vi "Pump Pause Selection.vi"(8 "error in (no error)":errorcluster, 11 "Pump Settings In":T1={"Output Device"=enum."Default", "Masterflex"={"VISA resource name"="", "Simulated?"=FALSE, "Pump Number"=0.0, "Reverse?"=FALSE}, "Ismatech"={"VISA resource name"="", "Simulated?"=FALSE, "Pump Number"=0.0, "Reverse?"=FALSE}, "Ismatech 3 Channel Settings"={"VISA resource name"="", "Pump Number"=1, "Channel Number"=0, "Simulated?"=TRUE, "Reverse?"=FALSE}, "VICI Settings"={"VISA resource name"="", "Pump ID"="", "Pump Head Vol"=0.0, "Reverse?"=FALSE, "Simulated?"=FALSE}, "Tacmina Settings"={"Analog DAQ Task"="", "Digital DAQ Task"=""}, "KNF SIMDOS Settings"={"VISA resource name"="", "Simulated?"=FALSE}, "ASIA Pump C"={"ASIA Pump #"=0, "channel"=0, "Simulated"=FALSE}, "FLOM Settings"={"VISA resource name"="", "Simulated?"=FALSE, "Pump Number"=0.0}, "SSI PR/LD Settings"={"VISA resource name"="", "Simulated?"=FALSE}, "SSI P40 Settings"={"VISA resource name"="", "Simulated?"=FALSE}, "Masterflex 75211 Settings"={"Analog DAQ Task"="", "Digital DAQ Task"=""}} {"Ismatech 3 Channel Settings"."Channel Number" min=0 max=3; "Ismatech 3 Channel Settings"."Pump Number" min=1; "Masterflex"."Pump Number" min=1.0 max=20.0 step=1.0; "Ismatech"."Pump Number" min=1.0 max=20.0 step=1.0; "ASIA Pump C"."channel" min=-1 max=1 step=1}) -> (0 "error out":errorcluster, 1 "Connection Error":bool, 3 "Pump Settings Out":T1={"Output Device"=enum."Default", "Masterflex"={"VISA resource name"="", "Simulated?"=FALSE, "Pump Number"=0.0, "Reverse?"=FALSE}, "Ismatech"={"VISA resource name"="", "Simulated?"=FALSE, "Pump Number"=0.0, "Reverse?"=FALSE}, "Ismatech 3 Channel Settings"={"VISA resource name"="", "Pump Number"=1, "Channel Number"=0, "Simulated?"=TRUE, "Reverse?"=FALSE}, "VICI Settings"={"VISA resource name"="", "Pump ID"="", "Pump Head Vol"=0.0, "Reverse?"=FALSE, "Simulated?"=FALSE}, "Tacmina Settings"={"Analog DAQ Task"="", "Digital DAQ Task"=""}, "KNF SIMDOS Settings"={"VISA resource name"="", "Simulated?"=FALSE}, "ASIA Pump C"={"ASIA Pump #"=0, "channel"=0, "Simulated"=FALSE}, "FLOM Settings"={"VISA resource name"="", "Simulated?"=FALSE, "Pump Number"=0.0}, "SSI PR/LD Settings"={"VISA resource name"="", "Simulated?"=FALSE}, "SSI P40 Settings"={"VISA resource name"="", "Simulated?"=FALSE}, "Masterflex 75211 Settings"={"Analog DAQ Task"="", "Digital DAQ Task"=""}} {"Ismatech 3 Channel Settings"."Channel Number" min=0 max=3; "Ismatech 3 Channel Settings"."Pump Number" min=1; "Masterflex"."Pump Number" min=1.0 max=20.0 step=1.0; "Ismatech"."Pump Number" min=1.0 max=20.0 step=1.0; "ASIA Pump C"."channel" min=-1 max=1 step=1})   [LabVIEW 2018, in "Pump Module.lvlib" / "Pump Module Engine.lvlib"]
uses:
  Pump Module Engine.lvlib
  Pump Settings Cluster.ctl
  Measure Instrument/PID 2 Output Enum.ctl
  Masterflex 7550-30/Controls/Settings Cluster.ctl
  Ismatec ISM 831C/Controls/Ismatech ISM831C Settings Cluster.ctl
  Ismatec 78001/Ismatec 4083.ctl
  VICI M50 Party Mode/Settings Cluster.ctl
  Tacmina QI/Tacmina QI DAQ Setting.ctl
  KNF Pump/Settings Cluster plus SIMDOS.ctl
  ASIA Pump/Pump Settings.ctl
  FLOM Pump/Settings Cluster.ctl
  SSI PR Class/SSI PR or LD Settings Cluster.ctl
  Masterflex 75211/Masterflex 75211 DAQ Setting.ctl
  Ismatec ISM 831C/Ismatec ISM 831C.lvlib
  Masterflex 7550-30/Masterflex 7550-30.lvlib
  VICI M50 Party Mode/VICI M6 M50 Party Mode.lvlib
  Tacmina QI/Tacmina QI.lvlib
  KNF Pump/KNF SIMDOS.lvlib
  ASIA Pump.lvlib
  FLOM Pump/FLOM Pump.lvlib
  SSI PR Class/SSI PR or LD Pump.lvlib
  Masterflex 75211/Masterflex 75211.lvlib
  SSI PR Class/SSI P40 Pump.lvlib
  Ismatec 78001/Ismatec 4308.lvlib
  Pump Module.lvlib
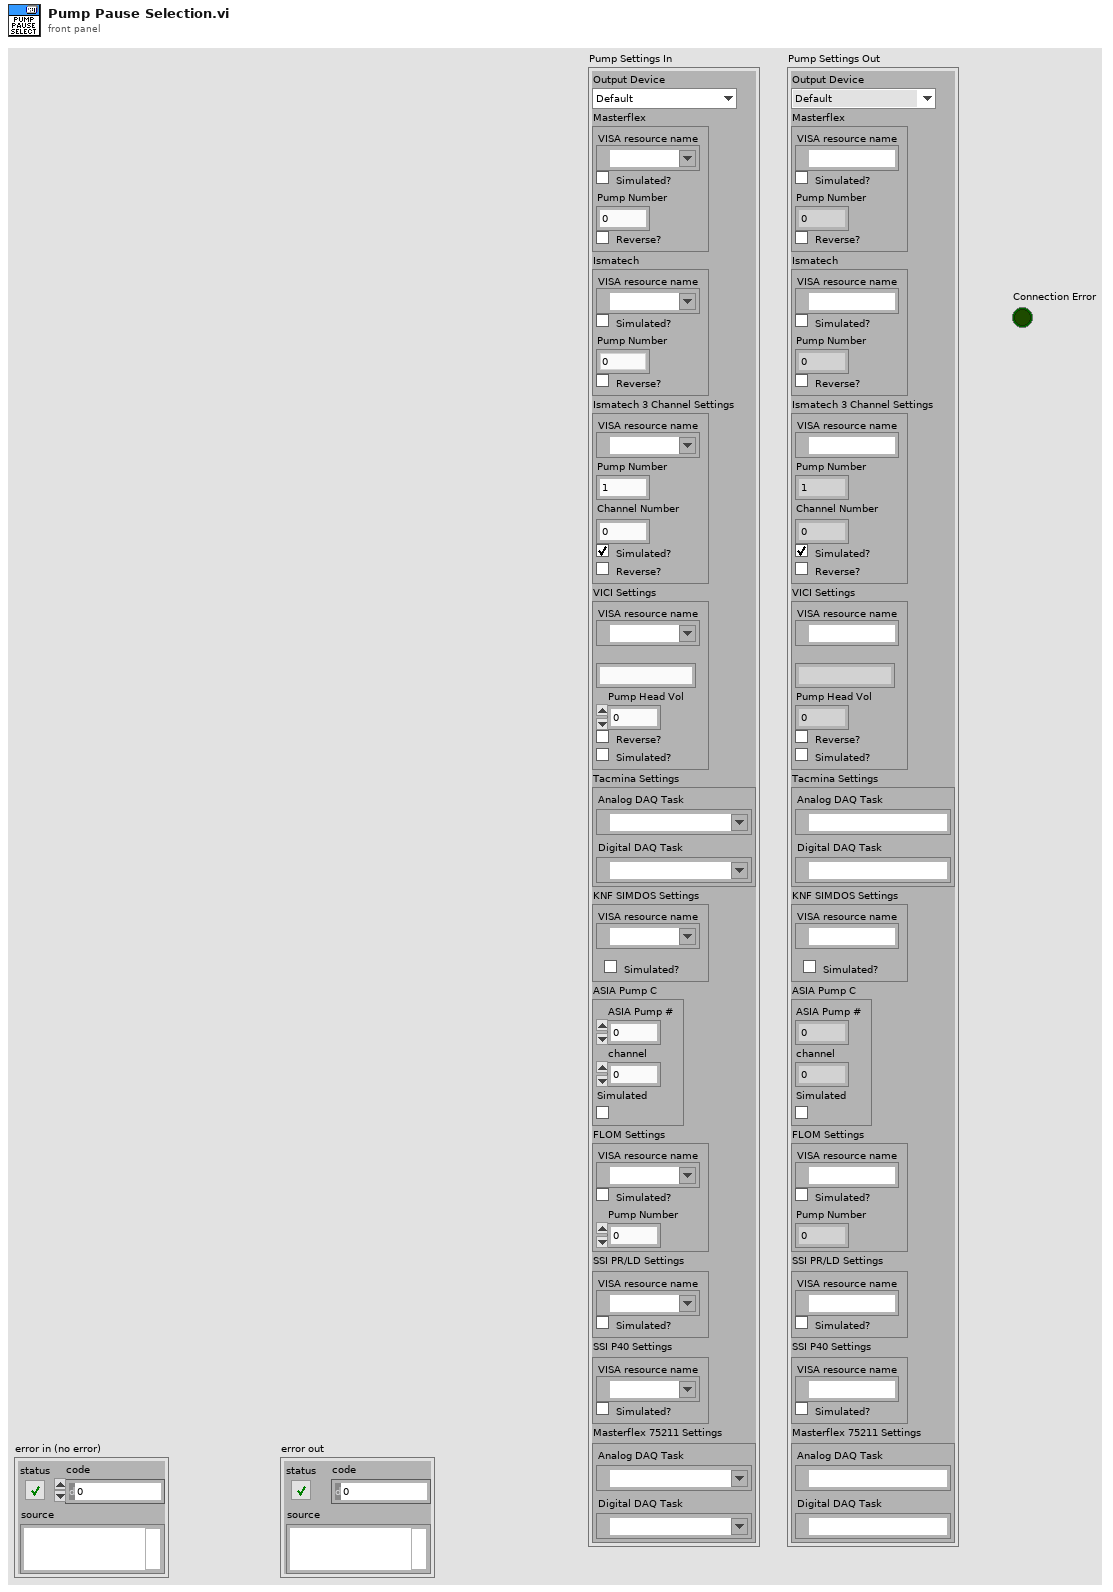
[diagram p1: front panel]
types:
  T1 = typedef "Pump Module.lvlib/Pump Settings Cluster.ctl" = cluster{"Output Device":T2, "Masterflex":T3, "Ismatech":T4, "Ismatech 3 Channel Settings":T5, "VICI Settings":T6, "Tacmina Settings":T7, "KNF SIMDOS Settings":T8, "ASIA Pump C":T9, "FLOM Settings":T10, "SSI PR/LD Settings":T11, "SSI P40 Settings":T11, "Masterflex 75211 Settings":T12}
  T2 = typedef "PID 2 Output Enum.ctl" = enum16{"Default", "Ismatec ISM 4308", "Ismatec ISM 831C", "Masterflex 7550-30", "VICI M6", "VICI M50", "Tacmina QI", "KNF SIMDOS", "ASIA Type C", "FLOM UI-22-11", "SSI PR/LD", "SSI P40", "Masterflex 75211-70"}
  T3 = typedef "Masterflex 7550-30.lvlib/Settings Cluster.ctl" = cluster{"VISA resource name":refnum<visa-resource-name>, "Simulated?":bool, "Pump Number":dbl, "Reverse?":bool}
  T4 = typedef "Ismatec ISM 831C.lvlib/Ismatech ISM831C Settings Cluster.ctl" = cluster{"VISA resource name":refnum<visa-resource-name>, "Simulated?":bool, "Pump Number":dbl, "Reverse?":bool}
  T5 = typedef "Ismatec 4308.lvlib/Ismatec 4083.ctl" = cluster{"VISA resource name":refnum<visa-resource-name>, "Pump Number":i16, "Channel Number":i16, "Simulated?":bool, "Reverse?":bool}
  T6 = typedef "VICI M6 M50 Party Mode.lvlib/Settings Cluster.ctl" = cluster{"VISA resource name":refnum<visa-resource-name>, "Pump ID":string, "Pump Head Vol":dbl, "Reverse?":bool, "Simulated?":bool}
  T7 = typedef "Tacmina QI.lvlib/Tacmina QI DAQ Setting.ctl" = cluster{"Analog DAQ Task":refnum<k21>, "Digital DAQ Task":refnum<k21>}
  T8 = typedef "KNF SIMDOS.lvlib/Settings Cluster plus SIMDOS.ctl" = cluster{"VISA resource name":refnum<visa-resource-name>, "Simulated?":bool}
  T9 = typedef "ASIA Pump.lvlib/Pump Settings.ctl" = cluster{"ASIA Pump #":i32, "channel":i32, "Simulated":bool}
  T10 = typedef "FLOM Pump.lvlib/Settings Cluster.ctl" = cluster{"VISA resource name":refnum<visa-resource-name>, "Simulated?":bool, "Pump Number":dbl}
  T11 = typedef "SSI PR or LD Pump.lvlib/SSI PR or LD Settings Cluster.ctl" = cluster{"VISA resource name":refnum<visa-resource-name>, "Simulated?":bool}
  T12 = typedef "Masterflex 75211.lvlib/Masterflex 75211 DAQ Setting.ctl" = cluster{"Analog DAQ Task":refnum<k21>, "Digital DAQ Task":refnum<k21>}
  T13 = typedef "SSI P40 Pump.lvlib/SSI P40 Settings Cluster.ctl" = cluster{"VISA resource name":refnum<visa-resource-name>, "Simulated?":bool}
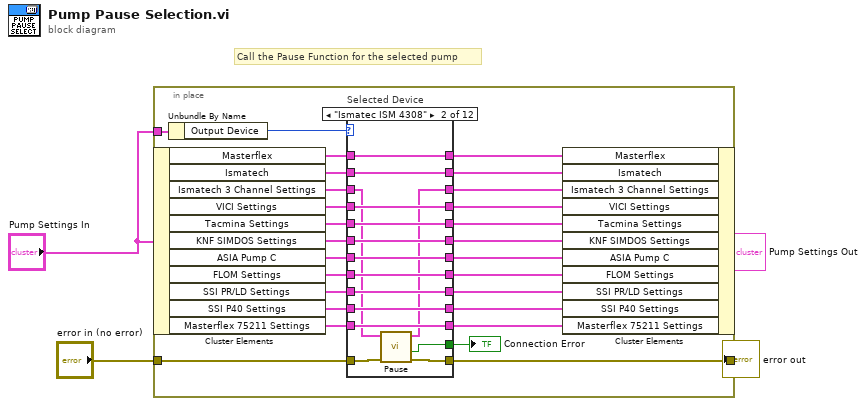
[diagram p0: block diagram]
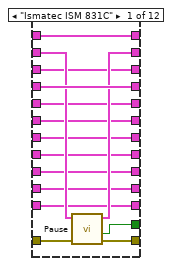
[diagram p2: hidden frame]
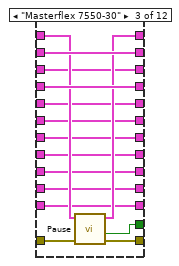
[diagram p3: hidden frame]
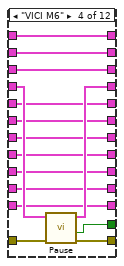
[diagram p4: hidden frame]
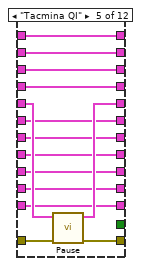
[diagram p5: hidden frame]
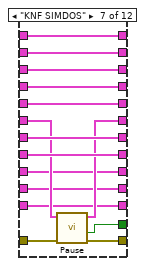
[diagram p7: hidden frame]
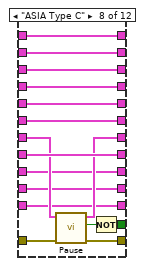
[diagram p8: hidden frame]
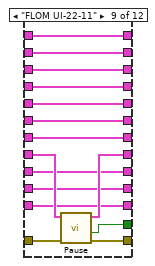
[diagram p9: hidden frame]
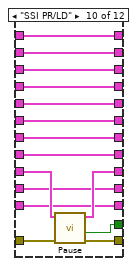
[diagram p10: hidden frame]
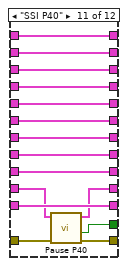
[diagram p11: hidden frame]
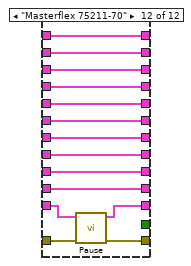
[diagram p12: hidden frame]
diagram:
  # "Call the Pause Function for the selected pump"
  n1 = in-place {
    in-place-border: "error in (no error)" -> [w31]
    in-place-border: [w30] -> w3
    in-place-border: "Pump Settings In" -> [w12]
    n2 = in-place-cluster #1("Pump Settings In") -> ("Masterflex"=w28:T3, "Ismatech"=w27:T4, "Ismatech 3 Channel Settings"=w5:T5, "VICI Settings"=w26:T6, "Tacmina Settings"=w25:T7, "KNF SIMDOS Settings"=w24:T8, "ASIA Pump C"=w23:T9, "FLOM Settings"=w22:T10, "SSI PR/LD Settings"=w21:T11, "SSI P40 Settings"=w7:T11, "Masterflex 75211 Settings"=w10:T12)
    n3 = Unbundle By Name(w12) -> ("Output Device"=w11:T2)
    n4 = case "Selected Device" shown="\"Ismatec ISM 4308\"" w11 {
      tunnel: w28 -> [w46 w61 w74 w90 w104 w117 w132 w148 w163 w178 w193 w207]
      tunnel: [w46 w61 w73 w90 w104 w117 w132 w148 w163 w178 w193 w207] -> w20
      tunnel: w27 -> [w44 w60 w76 w91 w105 w116 w131 w147 w162 w177 w192 w206]
      tunnel: [w42 w50 w72 w87 w100 w113 w125 w141 w156 w170 w183 w196] -> w30
      tunnel: [w43 w60 w76 w91 w105 w116 w131 w147 w162 w177 w192 w206] -> w19
      tunnel: w26 -> [w45 w59 w75 w89 w103 w115 w130 w146 w161 w176 w191 w205]
      tunnel: [w45 w59 w75 w88 w103 w115 w130 w146 w161 w176 w191 w205] -> w18
      tunnel: w25 -> [w40 w58 w70 w85 w102 w114 w129 w145 w160 w175 w190 w204]
      tunnel: [w40 w58 w70 w85 w101 w114 w129 w145 w160 w175 w190 w204] -> w17
      tunnel: w31 -> [w41 w51 w71 w86 w99 w113 w126 w142 w157 w171 w184 w197]
      tunnel: [w39 w57 w69 w84 w98 w112 w124 w144 w159 w174 w189 w203] -> w16
      tunnel: w24 -> [w39 w57 w69 w84 w98 w112 w123 w144 w159 w174 w189 w203]
      tunnel: [w38 w56 w68 w83 w97 w111 w128 w140 w158 w173 w188 w202] -> w15
      tunnel: w23 -> [w38 w56 w68 w83 w97 w111 w128 w139 w158 w173 w188 w202]
      tunnel: [w37 w55 w67 w82 w96 w110 w127 w143 w154 w172 w187 w201] -> w14
      tunnel: w22 -> [w37 w55 w67 w82 w96 w110 w127 w143 w155 w172 w187 w201]
      tunnel: [w36 w54 w66 w81 w95 w109 w122 w138 w153 w168 w186 w200] -> w13
      tunnel: w21 -> [w36 w54 w66 w81 w95 w109 w122 w138 w153 w169 w186 w200]
      tunnel: [w35 w49 w65 w80 _ _ w121 w136 w152 w167 w182 _] -> w29
      tunnel: w10 -> [w34 w53 w64 w79 w94 w108 w120 w135 w151 w166 w185 w199]
      tunnel: [w34 w53 w64 w79 w94 w108 w120 w135 w151 w166 w185 w198] -> w9
      tunnel: [w33 w52 w63 w78 w93 w107 w119 w134 w150 w165 w181 w195] -> w8
      tunnel: w7 -> [w33 w52 w63 w78 w93 w107 w119 w134 w150 w165 w180 w195]
      tunnel: [w32 w48 w62 w77 w92 w106 w118 w133 w149 w164 w179 w194] -> w6
      tunnel: w5 -> [w32 w47 w62 w77 w92 w106 w118 w133 w149 w164 w179 w194]
      frame "Ismatec ISM 831C" {
        n5 = call "Pause.vi"("error in (no error)"=w41, "Ismatech Settings In"=w44) -> ("error out"=w42:errorcluster, "Connection Error"=w35:bool, "Ismatech Settings Out"=w43:T4)  [unwired: 7 in]
      }
      frame "Ismatec ISM 4308" {
        n6 = call "Pause.vi"("error in (no error)"=w51, "Ismatech 3 Channel Settings In"=w47) -> ("error out"=w50:errorcluster, "Connection Error"=w49:bool, "Ismatech 3 Channel Settings Out"=w48:T5)  [unwired: 6 in, 1 out]
      }
      frame "Masterflex 7550-30" {
        n7 = call "Pause.vi"("error in (no error)"=w71, "Masterflex Settings in"=w74) -> ("error out"=w72:errorcluster, "Connection Error"=w65:bool, "Masterflex Settings out"=w73:T3)  [unwired: 7 in]
      }
      frame "VICI M6" {
        n8 = call "Pause.vi"("error in (no error)"=w86, "VICI Settings In"=w89) -> ("error out"=w87:errorcluster, "Connection Error"=w80:bool, "VICI Settings Out"=w88:T6)  [unwired: 7 in]
      }
      frame "Tacmina QI" {
        n9 = call "Pause.vi"("error in"=w99, "Tacmina Settings in"=w102) -> ("error out"=w100:errorcluster, "Tacmina Settings out"=w101:T7)  [unwired: 8 in]
      }
      frame "Default", Default {
      }
      frame "KNF SIMDOS" {
        n10 = call "Pause.vi"("error in (no error)"=w126, "KNF Settings In"=w123) -> ("error out"=w125:errorcluster, "Connection Error"=w121:bool, "KNF Settings Out"=w124:T8)  [unwired: 7 in]
      }
      frame "ASIA Type C" {
        n11 = call "Pause.vi"("error in (no error)"=w142, "ASIA Pump C Settings in"=w139) -> ("error out"=w141:errorcluster, "Task Completed"=w137:bool, "ASIA Pump C Settings out"=w140:T9)  [unwired: 7 in]
        n12 = Not(x=w137) -> (.not. x?=w136:bool)
      }
      frame "FLOM UI-22-11" {
        n13 = call "Pause.vi"("error in (no error)"=w157, "FLOM Settings in"=w155) -> ("error out"=w156:errorcluster, "Connection Error"=w152:bool, "FLOM Settings out"=w154:T10)  [unwired: 7 in]
      }
      frame "SSI PR/LD" {
        n14 = call "Pause.vi"("error in (no error)"=w171, "SSI PR Settings In"=w169) -> ("error out"=w170:errorcluster, "Connection Error"=w167:bool, "SSI PR Settings Out"=w168:T11)  [unwired: 6 in]
      }
      frame "SSI P40" {
        n15 = call "Pause P40.vi"("error in (no error)"=w184, "SSI P40 Settings In"=w180) -> ("error out"=w183:errorcluster, "Connection Error"=w182:bool, "SSI P40 Settings Out"=w181:T13)  [unwired: 7 in]
      }
      frame "Masterflex 75211-70" {
        n16 = call "Pause.vi"("error in"=w197, "Masterflex 75211 Settings"=w199) -> ("error out"=w196:errorcluster, "Masterflex 75211 Settings"=w198:T12)  [unwired: 8 in]
      }
    }
    "Connection Error" <- w29
    n17 = in-place-cluster #1("Masterflex"=w20, "Ismatech"=w19, "Ismatech 3 Channel Settings"=w6, "VICI Settings"=w18, "Tacmina Settings"=w17, "KNF SIMDOS Settings"=w16, "ASIA Pump C"=w15, "FLOM Settings"=w14, "SSI PR/LD Settings"=w13, "SSI P40 Settings"=w8, "Masterflex 75211 Settings"=w9) -> (→"Pump Settings Out":T1)
  }
  "error out" <- w3
